vi "List And Filter Controls From UI.vi"(8 "Error In":errorcluster, 11 "Appearance Actor In":refnum<class "Appearance Actor.lvclass">) -> (0 "Error Out":errorcluster, 3 "Appearance Actor Out":refnum<class "Appearance Actor.lvclass">)   [LabVIEW 2021, in "Appearance Actor.lvlib" / "Appearance Actor.lvclass"]
uses:
  Appearance Actor.lvclass
  Appearance Actor.lvclass/Appearance Actor.ctl
  Typedefs/Control Reference Lists--cluster.ctl
  Typedefs/Control Reference Lists-TitleBar--cluster.ctl
  Typedefs/Control Reference Lists-SideMenu--cluster.ctl
  Typedefs/Control Reference Lists-BodyPane--cluster.ctl
  Typedefs/Control Reference Lists-StatusBar--cluster.ctl
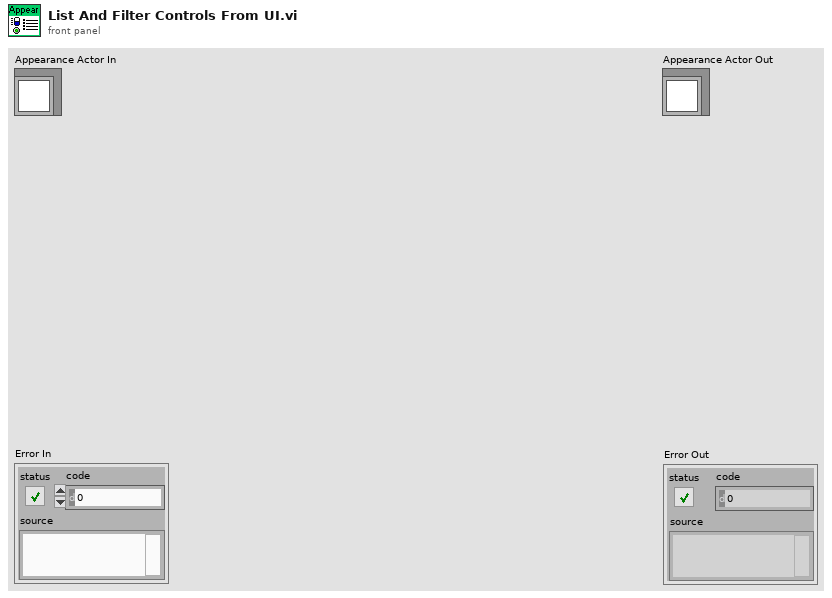
[diagram p1: front panel]
types:
  T1 = typedef "Appearance Actor.lvlib/Appearance Actor.lvclass/Control Reference Lists--cluster.ctl" = cluster{"TitleBar":T2, "SideMenu":T3, "BodyPane":T4, "StatusBar":T5}
  T2 = typedef "Appearance Actor.lvlib/Appearance Actor.lvclass/Control Reference Lists-TitleBar--cluster.ctl" = cluster{"Pane":refnum<vi>[], "Title":refnum<vi>, "Dark-CloseButton":refnum<vi>, "Light-CloseButton":refnum<vi>, "Dark-Buttons":refnum<vi>[], "Light-Buttons":refnum<vi>[], "Splitter":refnum<vi>}
  T3 = typedef "Appearance Actor.lvlib/Appearance Actor.lvclass/Control Reference Lists-SideMenu--cluster.ctl" = cluster{"Pane":refnum<vi>[], "Dark-Buttons":refnum<vi>[], "Light-Buttons":refnum<vi>[], "Splitter":refnum<vi>}
  T4 = typedef "Appearance Actor.lvlib/Appearance Actor.lvclass/Control Reference Lists-BodyPane--cluster.ctl" = cluster{"Pane":refnum<vi>[]}
  T5 = typedef "Appearance Actor.lvlib/Appearance Actor.lvclass/Control Reference Lists-StatusBar--cluster.ctl" = cluster{"Pane":refnum<vi>[], "Dark-Buttons":refnum<vi>[], "Light-Buttons":refnum<vi>[], "Splitter":refnum<vi>}
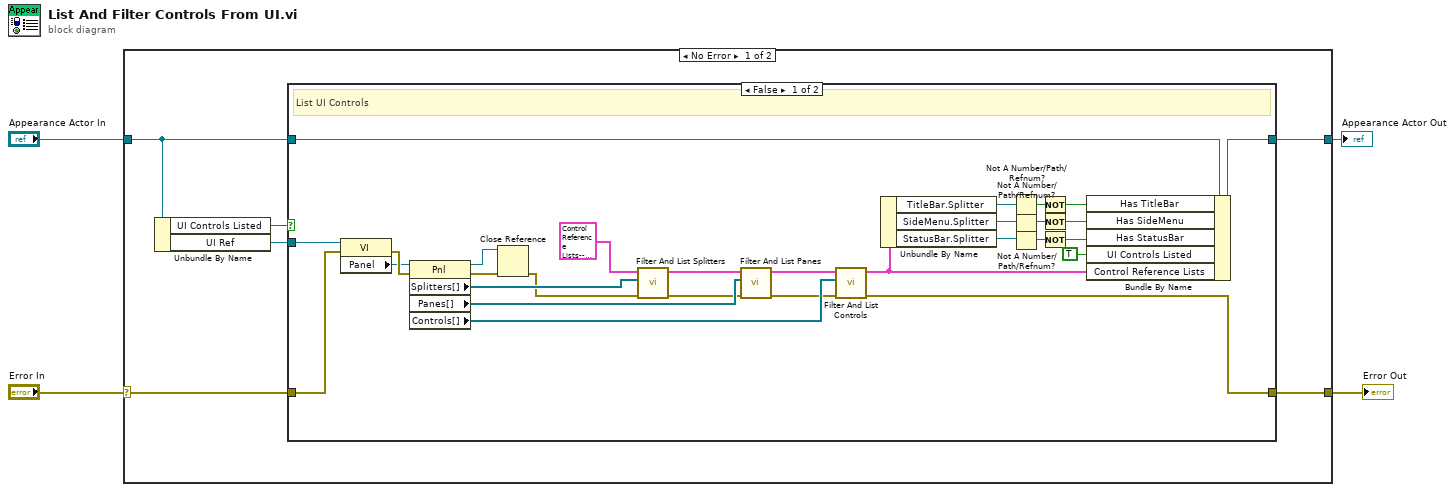
[diagram p0: block diagram]
diagram:
  n1 = case shown="No Error" "Error In" {
    selector: "Error In" -> [w10 w43]
    tunnel: [w8 w43] -> w3
    tunnel: "Appearance Actor In" -> [w7 w42]
    tunnel: [w9 w42] -> w1
    frame No Error {
      n2 = Unbundle By Name(w7) -> ("UI Controls Listed"=w6:bool, "UI Ref"=w5:refnum<vi>)
      n3 = case shown="False" w6 {
        tunnel: w5 -> [w39 _]
        tunnel: w10 -> [w37 w40]
        tunnel: w7 -> [w33 w41]
        tunnel: [w32 w41] -> w9
        tunnel: [w13 w40] -> w8
        frame False {
          # "List UI Controls"
          n4 = property class="VI"(reference=w39, error in=w37) -> (error out=w36:errorcluster, "Panel"=w35:refnum<vi>)  [unwired: 1 out]
          n5 = property class="Pnl"(reference=w35, error in=w36) -> (reference out=w38:refnum<vi>, error out=w34:errorcluster, "Splitters[]"=w30:refnum<vi>[], "Panes[]"=w25:refnum<vi>[], "Controls[]"=w29:refnum<vi>[])
          n6 = Close Reference(reference=w38, error in (no error)=w34) -> (error out=w28:errorcluster)
          n7 = call "Filter And List Splitters.vi"("Error In"=w28, "Splitter Refs"=w30, "Control Reference Lists In"=T1 {"TitleBar"={"Pane"=[], "Title"=refnum, "Dark-CloseButton"=refnum, "Light-CloseButton"=refnum, "Dark-Buttons"=[], "Light-Buttons"=[], "Splitter"=refnum}, "SideMenu"={"Pane"=[], "Dark-Buttons"=[], "Light-Buttons"=[], "Splitter"=refnum}, "BodyPane"={"Pane"=[]}, "StatusBar"={"Pane"=[], "Dark-Buttons"=[], "Light-Buttons"=[], "Splitter"=refnum}} ("Control Reference Lists")) -> ("Error Out"=w12:errorcluster, "Control Reference Lists Out"=w27:T1)  [unwired: 7 in]
          n8 = call "Filter And List Panes.vi"("Error In"=w12, "Splitter Refs"=w25, "Control Reference Lists In"=w27) -> ("Error Out"=w11:errorcluster, "Control Reference Lists Out"=w26:T1)  [unwired: 7 in]
          n9 = call "Filter And List Controls.vi"("Error In"=w11, "Control Refs"=w29, "Control Reference Lists In"=w26) -> ("Error Out"=w13:errorcluster, "Control Reference Lists Out"=w23:T1)  [unwired: 7 in]
          n10 = Unbundle By Name(w23) -> ("TitleBar.Splitter"=w22:refnum<vi>, "SideMenu.Splitter"=w18:refnum<vi>, "StatusBar.Splitter"=w15:refnum<vi>)
          n11 = Not A Number/Path/Refnum?(number/path/refnum=w22) -> (NaN/Path/Refnum?=w21:bool)
          n12 = Not A Number/Path/Refnum?(number/path/refnum=w18) -> (NaN/Path/Refnum?=w19:bool)
          n13 = Not A Number/Path/Refnum?(number/path/refnum=w15) -> (NaN/Path/Refnum?=w14:bool)
          n14 = Not(x=w21) -> (.not. x?=w20:bool)
          n15 = Not(x=w19) -> (.not. x?=w17:bool)
          n16 = Not(x=w14) -> (.not. x?=w16:bool)
          n17 = Bundle By Name(cluster=w33, "Has TitleBar"=w20, "Has SideMenu"=w17, "Has StatusBar"=w16, "UI Controls Listed"=TRUE ("UI Controls Registered"), "Control Reference Lists"=w23) -> (w32:refnum<class "Appearance Actor.lvclass">)
        }
        frame True {
          # "UI Controls Already Listed, Do Nothing"
        }
      }
    }
    frame Error {
    }
  }
  "Error Out" <- w3
  "Appearance Actor Out" <- w1
